vi "PathPlanner_PathFinder_Cost.vi"(9 "sGoal":T1, 11 "sStart":T1) -> (3 "Cost":dbl)   [LabVIEW 2019, in "PathPlanner24.lvlib"]
uses:
  PathPlanner24.lvlib
  TypeDef/PathPlannerFinderGridPosition.ctl
  PathPlanner_GridPosition_Get.vi
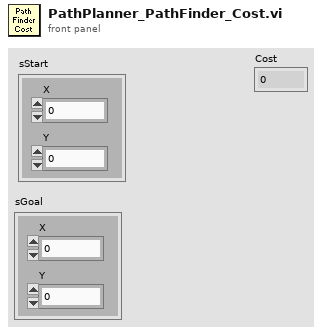
[diagram p1: front panel]
types:
  T1 = typedef "PathPlanner24.lvlib/PathPlannerFinderGridPosition.ctl" = cluster{"X":i32, "Y":i32}
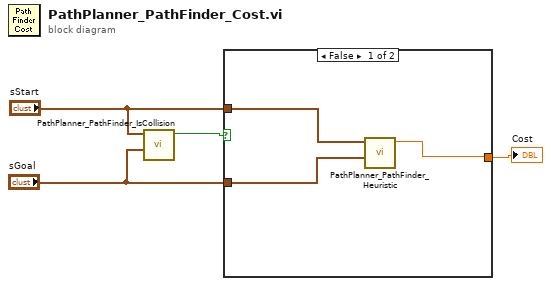
[diagram p0: block diagram]
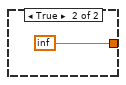
[diagram p2: hidden frame]
diagram:
  n1 = call "PathPlanner_PathFinder_IsCollision.vi"("sGoal"="sGoal", "sStart"="sStart") -> ("Collision"=w3:bool)  [unwired: 9 in]
  n2 = case shown="False" w3 {
    tunnel: [w5 inf] -> w4
    tunnel: "sStart" -> [w7 _]
    tunnel: "sGoal" -> [w6 _]
    frame False {
      n3 = call "PathPlanner_PathFinder_Heuristic.vi"("sGoal"=w6, "sStart"=w7) -> ("heuristic"=w5:dbl)  [unwired: 9 in]
    }
    frame True {
    }
  }
  "Cost" <- w4
